vi "InitWindow.vi"(8 "error in (no error)":errorcluster, 10 "This VI":refnum<vi>, 11 "DisplayWindow in":refnum<class "DisplayWindow.lvclass">) -> (0 "error out":errorcluster, 3 "DisplayWindow out":refnum<class "DisplayWindow.lvclass">)   [LabVIEW 2017, in "DisplayWindow.lvlib" / "DisplayWindow.lvclass"]
uses:
  DisplayWindow.lvclass
  DisplayWindow.lvclass/DisplayWindow.ctl
  <vilib>/Utility/miscctls.llb/LVPointTypeDef.ctl
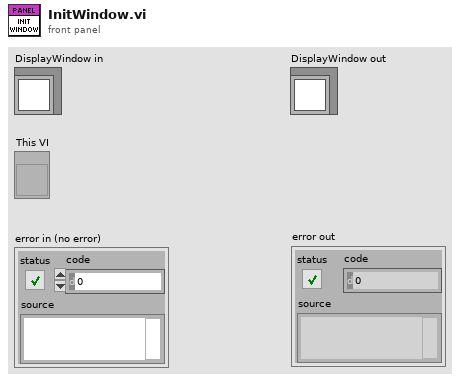
[diagram p1: front panel]
types:
  T1 = typedef "LVPointTypeDef.ctl" = cluster{"Horizontal":i16, "Vertical":i16}
  T2 = typedef "LVRectTypeDef.ctl" = cluster{"Left":i16, "Top":i16, "Right":i16, "Bottom":i16}
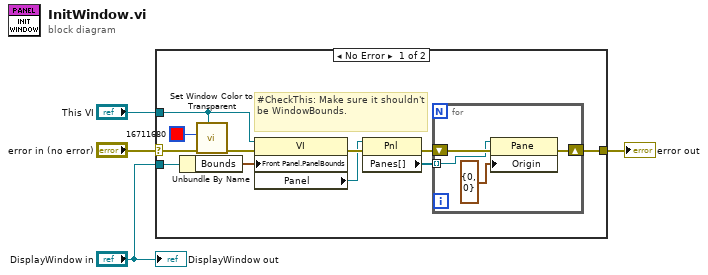
[diagram p0: block diagram]
diagram:
  n1 = case shown="No Error" "error in (no error)" {
    selector: "error in (no error)" -> [w8 w20]
    tunnel: "This VI" -> [w6 _]
    tunnel: [w10 w20] -> w3
    tunnel: "DisplayWindow in" -> [w9 _]
    frame No Error {
      # "#CheckThis: Make sure it shouldn't be WindowBounds."
      n2 = Unbundle By Name(w9) -> ("Bounds"=w11:T2)
      n3 = call "Set Window Color to Transparent.vi"("Calling VI's reference"=w6, "error in (no error)"=w8, "Color to Replace"=u32 16711680) -> ("error out"=w7:errorcluster)  [unwired: 5 in]
      n4 = property class="VI"(reference=w6, error in=w7, "Front Panel.PanelBounds"=w11) -> (error out=w13:errorcluster, "Panel"=w12:refnum<vi>)  [unwired: 1 out]
      n5 = property class="Pnl"(reference=w12, error in=w13) -> (error out=w15:errorcluster, "Panes[]"=w14:refnum<vi>[])  [unwired: 1 out]
      n6 = for {
        tunnel: w14 -> [w17] mode=indexing
        shift-right: [w19] -> w10
        shift-left: w15 -> [w18]
        n7 = property class="Pane"(reference=w17, error in=w18, "Origin"=T1 {"Horizontal"=0, "Vertical"=0}) -> (error out=w19:errorcluster)  [unwired: 1 out]
      }
    }
    frame Error {
    }
  }
  "error out" <- w3
  "DisplayWindow out" <- "DisplayWindow in"
